vi "TIO Device Tick.vi"(8 "Error in":errorcluster, 10 "TIO State":T2={"Awaiting REP"=FALSE, "REQ ID"=500, "dstreams in"=[], "pstreams"=[], "timebases"=[]}, 11 "TIO":T3={"TS Connection"={"Type"=enum."TCP", "Serial"="serial:///dev/cu.usbserial-00000", "TCP"=refnum, "Timeout"=500}, "REQ"=refnum, "REP"=refnum}) -> (0 "Error out":errorcluster={"status"=TRUE, "code"=-1073807252, "source"="VISA Read in SLIP Decode Serial Read.vi->NN VISA Read.vi->NN RPC.vi"}, 1 "Data Out":T1, 2 "TIO State":T2={"Awaiting REP"=FALSE, "REQ ID"=500, "dstreams in"=[], "pstreams"=[], "timebases"=[]}, 3 "TIO Out":T3={"TS Connection"={"Type"=enum."TCP", "Serial"="serial:///dev/cu.usbserial-00000", "TCP"=refnum, "Timeout"=500}, "REQ"=refnum, "REP"=refnum})   [LabVIEW 2017]
uses:
  <instrlib>/tio-labview/TIO Library/TIO Stream Write.vi
  <instrlib>/tio-labview/TIO Library/TIO RPC Form Request.vi
  <instrlib>/tio-labview/TIO Library/TIO SLIP Serial Write.vi
  <instrlib>/tio-labview/TIO Library/TIO Form Packet.vi
  <instrlib>/tio-labview/TIO Library/TIO SLIP Encode.vi
  <instrlib>/tio-labview/TIO Library/TIO Serial Checksum CRC32.vi
panel:
  out "Last Log":string
  # "TIO Tick"
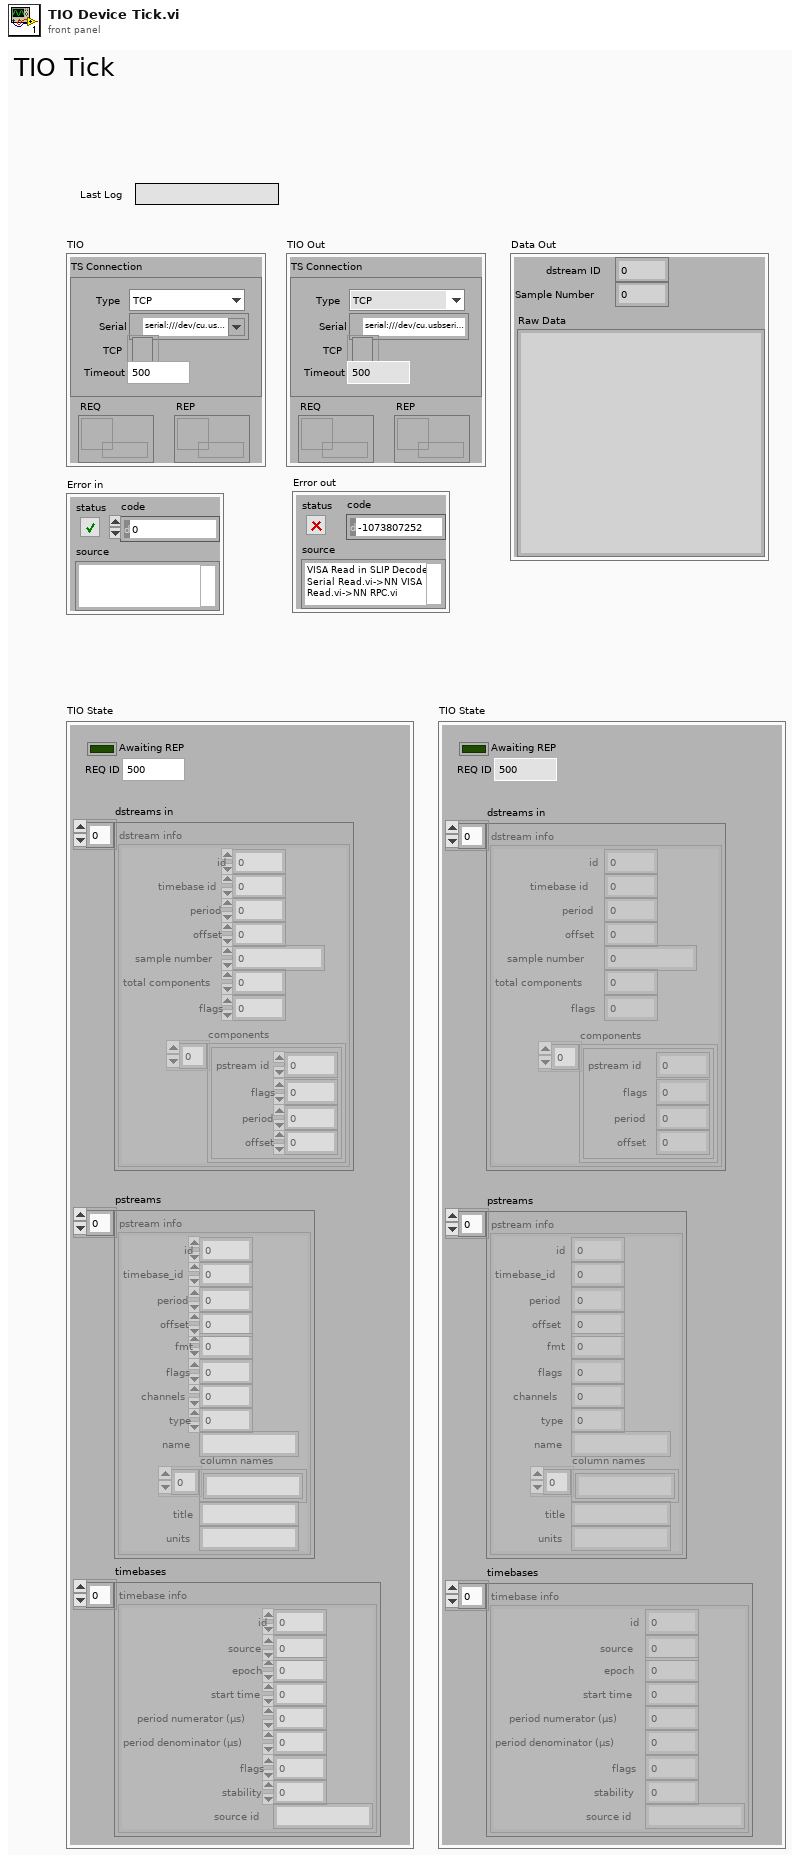
[diagram p1: front panel]
types:
  T1 = cluster{"dstream ID":u16, "Sample Number":u32, "Raw Data":string}
  T2 = cluster{"Awaiting REP":bool, "REQ ID":u32, "dstreams in":cluster{"id":u16, "timebase id":u16, "period":u32, "offset":u32, "sample number":u64, "total components":u16, "flags":u16, "components":cluster{"pstream id":u16, "flags":u16, "period":u32, "offset":u32}[]}[], "pstreams":cluster{"id":u16, "timebase_id":u16, "period":u32, "offset":u32, "fmt":i32, "flags":u16, "channels":u16, "type":u8, "name":string, "column names":string[], "title":string, "units":string}[], "timebases":cluster{"id":u16, "source":u16, "epoch":u32, "start time":u32, "period numerator (µs)":i32, "period denominator (µs)":u16, "flags":u16, "stability":u8, "source id":string}[]}
  T3 = cluster{"TS Connection":cluster{"Type":enum16{"TCP", "Serial"}, "Serial":refnum<visa-resource-name>, "TCP":refnum<k5>, "Timeout":u32}, "REQ":refnum<queue>, "REP":refnum<queue>}
  T4 = cluster{"Type":enum16{"TCP", "Serial"}, "Serial":refnum<visa-resource-name>, "TCP":refnum<k5>, "Timeout":u32}
  T5 = enum16{"big-endian, network order", "native, host order", "little-endian"}
  T6 = cluster{"id":u16, "source":u16, "epoch":u32, "start time":u32, "period numerator (µs)":i32, "period denominator (µs)":u16, "flags":u16, "stability":u8, "source id":string}[]
  T7 = cluster{"id":u16, "timebase_id":u16, "period":u32, "offset":u32, "fmt":i32, "flags":u16, "channels":u16, "type":u8, "name":string, "column names":string[], "title":string, "units":string}[]
  T8 = cluster{"id":u16, "timebase_id":u16, "period":u32, "offset":u32, "fmt":i32, "flags":u16, "channels":u16, "type":u8, "name":string, string[], "title":string, "units":string}[]
  T9 = cluster{"id":u16, "timebase id":u16, "period":u32, "offset":u32, "sample number":u64, "total components":u16, "flags":u16, "components":cluster{"pstream id":u16, "flags":u16, "period":u32, "offset":u32}[]}[]
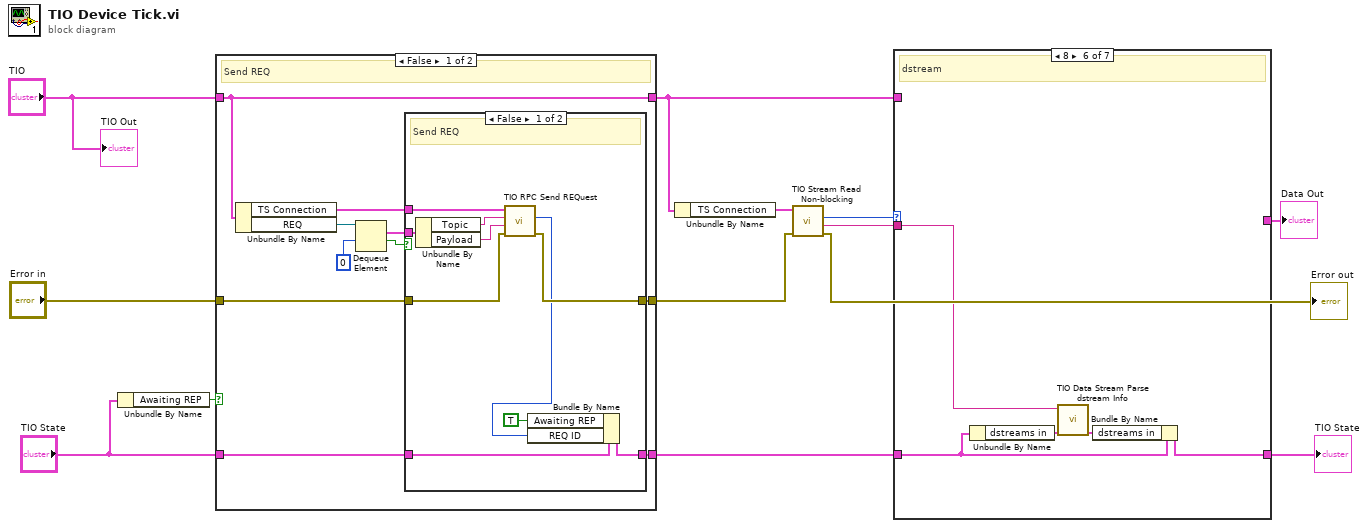
[diagram p0: block diagram]
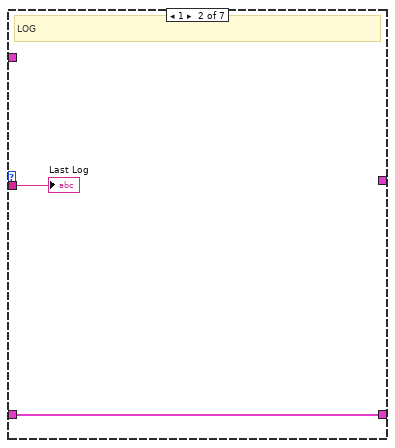
[diagram p3: hidden frame]
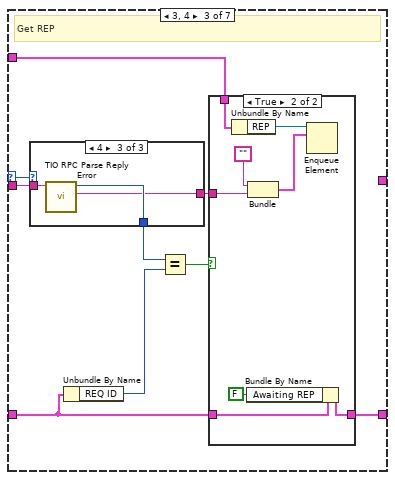
[diagram p4: hidden frame]
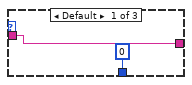
[diagram p5: hidden frame]
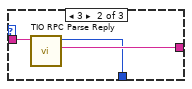
[diagram p6: hidden frame]
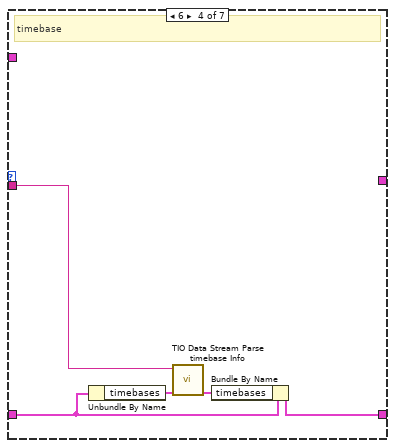
[diagram p8: hidden frame]
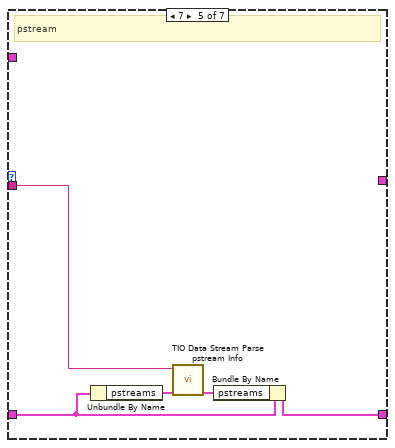
[diagram p9: hidden frame]
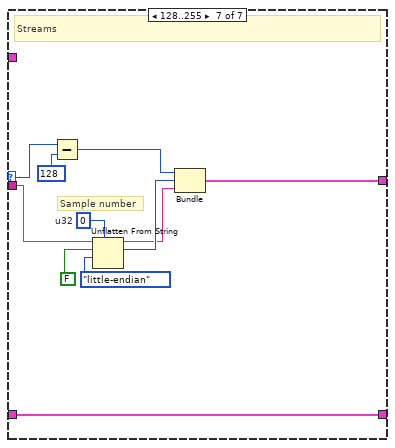
[diagram p10: hidden frame]
diagram:
  n1 = Unbundle By Name("TIO State") -> ("Awaiting REP"=w7:bool)
  n2 = case shown="False" w7 {
    tunnel: [w23 w36] -> w10
    tunnel: [w19 w38] -> w5
    tunnel: "TIO" -> [w19 w38]
    tunnel: "TIO State" -> [w15 w37]
    tunnel: [w16 w37] -> w6
    tunnel: "Error in" -> [w14 w36]
    frame False {
      # "Send REQ"
      n3 = Unbundle By Name(w19) -> ("TS Connection"=w18:T4, "REQ"=w17:refnum<queue>)
      n4 = Dequeue Element(queue=w17, timeout in ms (-1)=0) -> (element=w21:cluster{"Topic":string, "Payload":string}, timed out?=w20:bool)  [unwired: 1 in, 2 out]
      n5 = case shown="False" w20 {
        tunnel: [w33 w34] -> w23
        tunnel: w18 -> [w32 _]
        tunnel: w21 -> [w30 _]
        tunnel: [w27 w35] -> w16
        tunnel: w15 -> [w28 w35]
        tunnel: w14 -> [w25 w34]
        frame False {
          # "Send REQ"
          n6 = Unbundle By Name(w30) -> ("Topic"=w29:string, "Payload"=w31:string)
          n7 = call <instrlib>:"TIO RPC Send REQuest.vi"("error in (no error)"=w25, "Payload"=w31, "Topic"=w29, "TS Connection"=w32) -> ("error out"=w33:errorcluster, "Request ID"=w24:u16)  [unwired: 5 in, 1 out]
          n8 = Bundle By Name(cluster=w28, "Awaiting REP"=TRUE, "REQ ID"=w24) -> (w27:T2)
        }
        frame True {
          # "REQ Notification timeout"
        }
      }
    }
    frame True {
      # "Awaiting REP"
    }
  }
  n9 = Unbundle By Name(w5) -> ("TS Connection"=w4:T4)
  n10 = call <instrlib>:"TIO Stream Read Non-blocking.vi"("error in (no error)"=w10, "TS Connection"=w4) -> ("error out"=→"Error out":errorcluster, "Payload"=w8:string, "Type"=w9:u16)  [unwired: 6 in, 1 out]
  n11 = case shown="8" w9 {
    selector: w9 -> [_ _ w42 _ _ _ w93]
    tunnel: w8 -> [_ w41 w50 w70 w75 w82 w85]
    tunnel: w5 -> [_ _ w43 _ _ _ _]
    tunnel: [w39 w40 w44 w71 w76 w80 w91] -> w2
    tunnel: w6 -> [w39 w40 w45 w72 w77 w81 w91]
    tunnel: [_ _ _ _ _ _ w89] -> w1
    frame 0, Default {
    }
    frame 1 {
      # "LOG"
      "Last Log" <- w41
    }
    frame 3, 4 {
      # "Get REP"
      n12 = case shown="4" w42 {
        tunnel: w50 -> [w52 w55 w58]
        tunnel: [w52 w54 w56] -> w49
        tunnel: [u16 0 ("Request ID") w53 w57] -> w47
        frame Default {
        }
        frame 3 {
          n13 = call <instrlib>:"TIO RPC Parse Reply.vi"("Payload"=w55) -> ("Payload"=w54:string, "Request ID"=w53:u16)  [unwired: 9 in]
        }
        frame 4 {
          n14 = call <instrlib>:"TIO RPC Parse Reply Error.vi"("Payload"=w58) -> ("Payload"=w56:string, "Request ID"=w57:u16)  [unwired: 8 in, 1 out]
        }
      }
      n15 = Unbundle By Name(w45) -> ("REQ ID"=w46:u32)
      n16 = Equal?(x=w47, y=w46) -> (x = y?=w48:bool)
      n17 = case shown="True" w48 {
        tunnel: w49 -> [_ w62]
        tunnel: w45 -> [w59 w67]
        tunnel: [w59 w66] -> w44
        tunnel: w43 -> [_ w65]
        frame False {
        }
        frame True {
          n18 = Unbundle By Name(w65) -> ("REP"=w64:refnum<queue>)
          n19 = Bundle By Name(cluster=w67, "Awaiting REP"=FALSE) -> (w66:T2)
          n20 = Bundle("", "Payload"=w62) -> (w63:cluster{string, "Payload":string})  [unwired: 1 in]
          n21 = Enqueue Element(queue=w64, element=w63) -> ()  [unwired: 2 in, 3 out]
        }
      }
    }
    frame 6 {
      # "timebase"
      n22 = Unbundle By Name(w72) -> ("timebases"=w69:T6)
      n23 = call <instrlib>:"TIO Data Stream Parse timebase Info.vi"("timebases in"=w69, "timebase info raw"=w70) -> ("timebases out"=w68:T6)  [unwired: 8 in, 1 out]
      n24 = Bundle By Name(cluster=w72, "timebases"=w68) -> (w71:T2)
    }
    frame 7 {
      # "pstream"
      n25 = Unbundle By Name(w77) -> ("pstreams"=w74:T7)
      n26 = call <instrlib>:"TIO Data Stream Parse pstream Info.vi"("pstreams in"=w74, "pstream info raw"=w75) -> ("pstreams out"=w73:T8)  [unwired: 9 in]
      n27 = Bundle By Name(cluster=w77, "pstreams"=w73) -> (w76:T2)
    }
    frame 8 {
      # "dstream"
      n28 = Unbundle By Name(w81) -> ("dstreams in"=w79:T9)
      n29 = call <instrlib>:"TIO Data Stream Parse dstream Info.vi"("dstreams in"=w79, "dstream info raw"=w82) -> ("dstreams in"=w78:T9)  [unwired: 8 in, 1 out]
      n30 = Bundle By Name(cluster=w81, "dstreams in"=w78) -> (w80:T2)
    }
    frame 128..255 {
      w86 = u32 0  # u32
      # "Sample number"
      # "Streams"
      n31 = Subtract(x=w93, y=u16 128) -> (x-y=w90:u16)
      n32 = Unflatten From String(type=w86, binary string=w85, data includes array or string size? (T)=FALSE, byte order (0:big-endian, network order)=T5."little-endian") -> (rest of the binary string=w83:string, value=w84:u32)  [unwired: 1 in, 1 out]
      n33 = Bundle(w90, "u32"=w84, w83) -> (w89:cluster{u16, "u32":u32, string})  [unwired: 1 in]
    }
  }
  "TIO State" <- w2
  "Data Out" <- w1
  "TIO Out" <- "TIO"
